vi "Test_R_S.vi"() -> ()   [LabVIEW 2023, in "R_S.lvlib"]
uses:
  R_S.lvlib
panel:
  out "EVM_ALL_Carrier_Mean":string
  out "PPDU_Power_Mean":string
  out "error out":errorcluster
  out "Response":string
  in  "VISA_CMD":string="SYST:PRES"
  in  "VISA in":refnum<visa-resource-name>="TCPIP::20020-100136::inst0::INSTR"
  # "TCPIP::Vince_Wu-NB::inst0::INSTR"
  # "TCPIP0::192.168.88.12::inst0::INSTR"
  # "TCPIP::cmp20020-100136::hislip0::INSTR"
  # "TCPIP::192.168.88.12::hislip0::INSTR"
  # "*IDN?"
  # "FETCh:WLAN:MEAS:MEValuation:TRACe:EVMagnitude:SYMBol:AVERage?"
  # "SYST:ERR?"
  # "FETCh:BURSt:ALL:FORMatted?"
  # "FETCh:BURSt:PPDU:EVM:ALL:AVERage?\nFETCh:WLAN:MEAS:MEValuation:TRACe:EVMagnitude:SYMBol:AVERage?"
  # "FETCh:BURSt:PPDU:EVM:ALL:AVERage?"
  # "FETC:BURS:ALL:FORM?"
  # "FETCh:BURSt:ALL:FORMatted?"
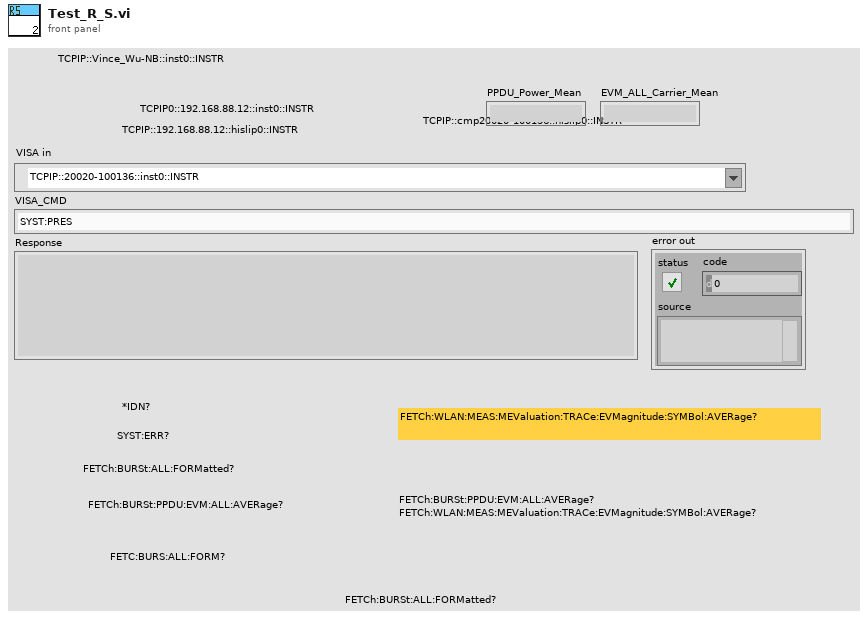
[diagram p1: front panel]
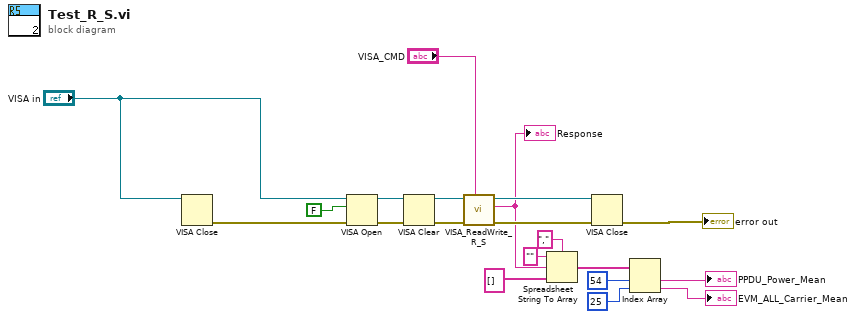
[diagram p0: block diagram]
diagram:
  n1 = VISA Close(VISA resource name="VISA in") -> (error out=w16:errorcluster)  [unwired: 1 in]
  n2 = VISA Open(duplicate session (F)=FALSE, error in (no error)=w16, VISA resource name="VISA in") -> (VISA resource name=w17:refnum<visa-resource-name>, error out=w18:errorcluster)  [unwired: 2 in]
  n3 = VISA Clear(VISA resource name=w17, error in (no error)=w18) -> (VISA resource name out=w14:refnum<visa-resource-name>, error out=w15:errorcluster)
  n4 = call "VISA_ReadWrite_R_S.vi"("VISA_CMD"="VISA_CMD", "error in"=w15, "VISA in"=w14) -> ("error out"=w12:errorcluster, "Response"=w9:string, "VISA out"=w10:refnum<visa-resource-name>)  [unwired: 6 in]
  "Response" <- w9
  n5 = Spreadsheet String To Array(delimiter (Tab)=",", format string="", spreadsheet string=w9, array type (2D Dbl)=string[] []) -> (array=w6:string[])
  n6 = VISA Close(VISA resource name=w10, error in (no error)=w12) -> (error out=→"error out":errorcluster)
  n7 = Index Array(array=w6, index #1=54 ("index"), index #2=25 ("index")) -> (element #1=→"PPDU_Power_Mean":string, element #2=→"EVM_ALL_Carrier_Mean":string)
